vi "Close Connection.vi"(8 "error in (no error)":errorcluster, 11 "TCPIP in":refnum<class "TCPIP.lvclass">) -> (0 "error out":errorcluster, 3 "TCPIP out":refnum<class "TCPIP.lvclass">)   [LabVIEW 2018, in "TCPIP.lvclass"]
uses:
  TCPIP.lvclass
  TCPIP.lvclass/TCPIP.ctl
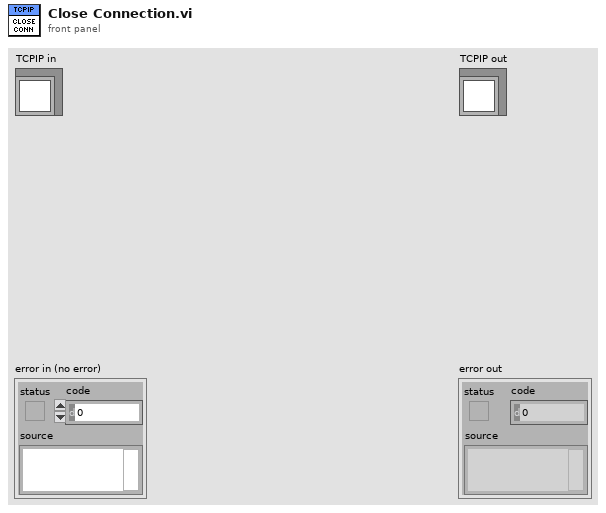
[diagram p1: front panel]
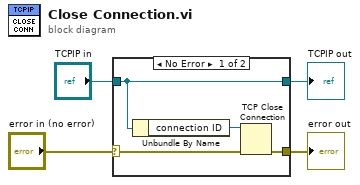
[diagram p0: block diagram]
diagram:
  n1 = case shown="No Error" "error in (no error)" {
    selector: "error in (no error)" -> [w8 w10]
    tunnel: [w7 w10] -> w3
    tunnel: [w6 w9] -> w1
    tunnel: "TCPIP in" -> [w6 w9]
    frame No Error {
      n2 = Unbundle By Name(w6) -> ("connection ID"=w5:refnum<k5>)
      n3 = TCP Close Connection(connection ID=w5, error in (no error)=w8) -> (error out=w7:errorcluster)  [unwired: 1 in, 1 out]
    }
    frame Error {
    }
  }
  "error out" <- w3
  "TCPIP out" <- w1
